vi "Ensenso_Receiver.vi"() -> ()   [LabVIEW 2015]
uses:
  <vilib>/Utility/tcp.llb/UDP Multicast Read-Write Open.vi
panel:
  out "error out":errorcluster
  in  "Stop":bool
  out "ROS Time":dbl
  out "x":dbl
  out "Seq No":dbl
  out "Translation":dbl[][](graph)
  out "y":dbl
  out "z":dbl
  out "pitch":dbl
  out "Rotation":dbl[][](graph)
  out "yaw":dbl
  out "POSE":dbl[](array[numeric])
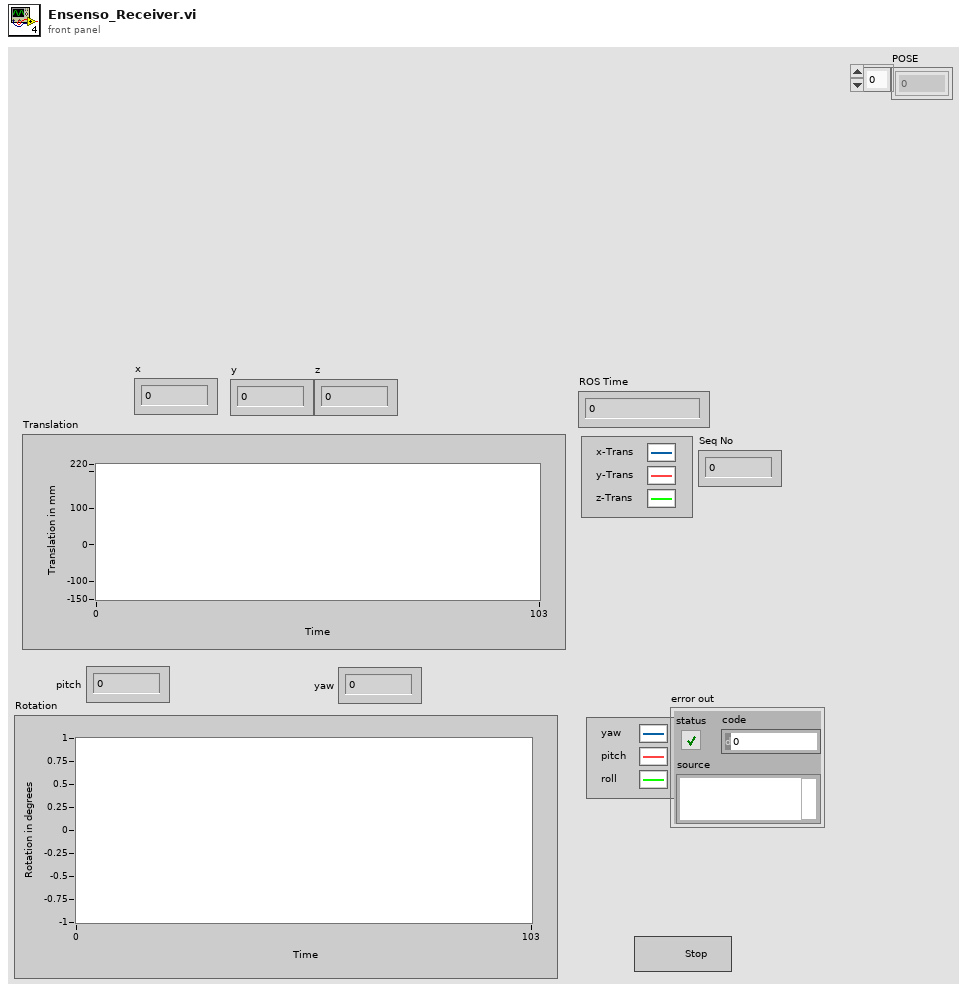
[diagram p1: front panel]
types:
  T1 = cluster{"array type (2D Dbl)[0]":dbl, "array type (2D Dbl)[1]":dbl, "array type (2D Dbl)[2]":dbl, "array type (2D Dbl)[3]":dbl, "array type (2D Dbl)[4]":dbl, "array type (2D Dbl)[5]":dbl, "array type (2D Dbl)[6]":dbl, "array type (2D Dbl)[7]":dbl, "array type (2D Dbl)[8]":dbl}
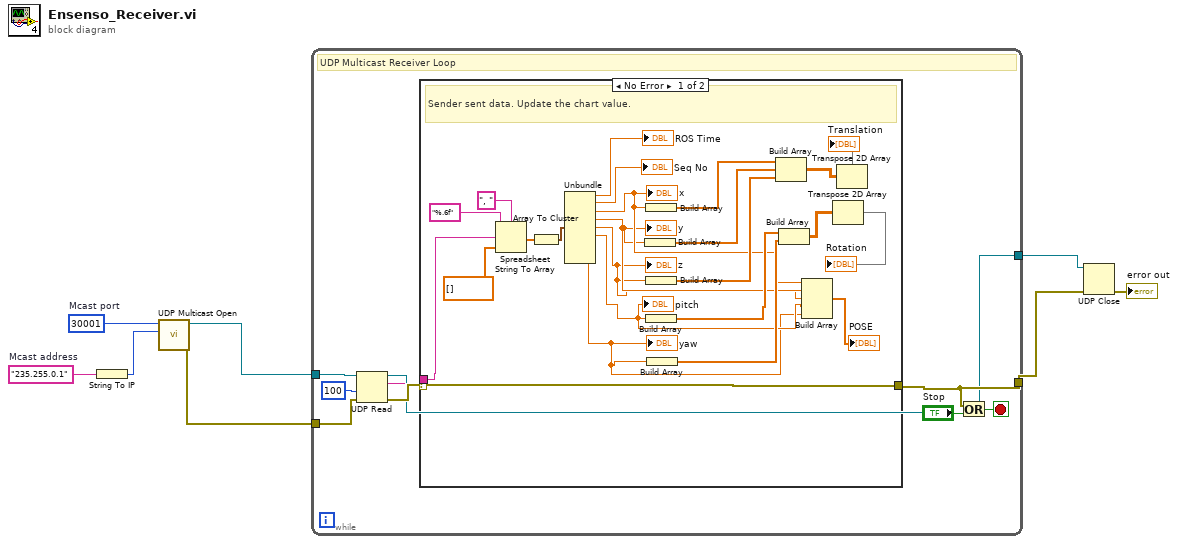
[diagram p0: block diagram]
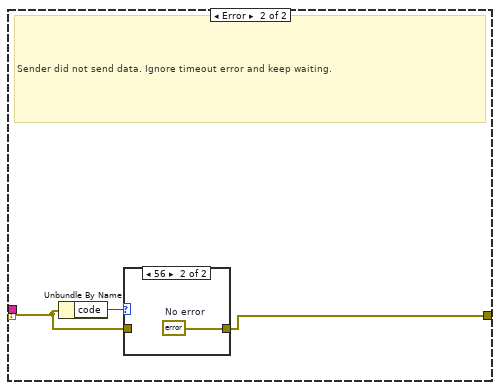
[diagram p2: hidden frame]
diagram:
  w3 = u16 30001  # Mcast port
  w7 = "235.255.0.1"  # Mcast address
  n1 = String To IP(1:w7) -> (0:w2:u32)
  n2 = call-poly <vilib>:"UDP Multicast Open.vi"("multicast addr"=w2, "port"=w3) -> ("error out"=w5:errorcluster, "connection ID"=w4:refnum<k16>)  [unwired: 7 in, 1 out]
  n3 = while {
    tunnel: w4 -> [w17]
    tunnel: [w10] -> w8
    tunnel: w5 -> [w14]
    tunnel: [w11] -> w6
    stop <- w15 stop-if-true
    # "UDP Multicast Receiver Loop"
    n4 = UDP Read(connection ID=w17, timeout ms (25000)=100, 8:w14) -> (data out=w9:string, error out=w12:errorcluster, 3:w10:refnum<k16>)  [unwired: 3 out]
    n5 = case shown="No Error" w12 {
      selector: w12 -> [w41 w43]
      tunnel: w9 -> [w30 _]
      tunnel: [w41 w42] -> w11
      frame No Error {
        # "Sender sent data. Update the chart value."
        n6 = Spreadsheet String To Array(delimiter (Tab)=", ", format string="%.6f", spreadsheet string=w30, array type (2D Dbl)=dbl[] []) -> (array=w28:dbl[])
        n7 = Array To Cluster(array=w28) -> (cluster=w29:T1)
        n8 = Unbundle(w29) -> ("array type (2D Dbl)[0]"=→"ROS Time":dbl, "array type (2D Dbl)[1]"=→"Seq No":dbl, "array type (2D Dbl)[2]"=w23:dbl, "array type (2D Dbl)[3]"=w22:dbl, "array type (2D Dbl)[4]"=w21:dbl, "array type (2D Dbl)[5]"=w20:dbl, "array type (2D Dbl)[6]"=w19:dbl)  [unwired: 2 out]
        "x" <- w23
        "y" <- w22
        "z" <- w21
        "pitch" <- w20
        "yaw" <- w19
        n9 = Build Array(w22) -> (w37:dbl[])
        n10 = Build Array(w23) -> (w24:dbl[])
        n11 = Build Array(w21) -> (w25:dbl[])
        n12 = Build Array(w20) -> (w35:dbl[])
        n13 = Build Array(w19) -> (w34:dbl[])
        n14 = Build Array(w24, w37, w25) -> (w36:dbl[][])
        n15 = Build Array(w35, w34) -> (w39:dbl[][])
        n16 = Build Array(w23, w22, w21, w20, w19) -> (→"POSE":dbl[])
        n17 = Transpose 2D Array(2D array=w39) -> (transposed array=→"Rotation":dbl[][])
        n18 = Transpose 2D Array(2D array=w36) -> (transposed array=→"Translation":dbl[][])
      }
      frame Error {
        # "Sender did not send data. Ignore timeout error and keep waiting."
        n19 = Unbundle By Name(w43) -> ("code"=w44:i32)
        n20 = case shown="56" w44 {
          tunnel: w43 -> [w45 _]
          tunnel: [w45 w46] -> w42
          frame Default {
          }
          frame 56 {
            w46 = errorcluster {"status"=FALSE, "code"=0, "source"=""}  # No error
          }
        }
      }
    }
    n21 = Or(x=w11, y="Stop") -> (x .or. y?=w15:bool)
  }
  n22 = UDP Close(connection ID=w8, 8:w6) -> (error out=→"error out":errorcluster)  [unwired: 1 out]
